vi "TagBus_Initialize_Map Data Type.vi"(11 "Value":variant) -> (3 "data type":T1)   [LabVIEW 2015, in "TagBus.lvclass"]
uses:
  TagBus.lvclass
  <vilib>/NI/Tag Bus/tag/Data Type.ctl
  <vilib>/Utility/Data Type/NI_Data Type.lvlib
  <vilib>/NI/Tag Bus/tag/tag descriptor.lvclass
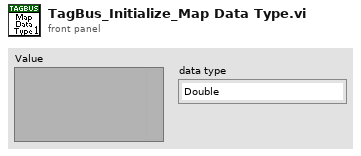
[diagram p1: front panel]
types:
  T1 = typedef "tag bus.lvlib/tag descriptor.lvclass/Data Type.ctl" = enum16{"Double", "Single", "I64", "I32", "I16", "I8", "U64", "U32", "U16", "U8", "Boolean", "String", "Array of Double", "Array of Single", "Array of I64", "Array of I32", "Array of I16", "Array of I8", "Array of U64", "Array of U32", "Array of U16", "Array of U8", "Array of Boolean", "Array of String"}
  T2 = typedef "NI_Data Type.lvlib/Data Type.ctl" = enum8{"Invalid Type", "Void", "I8", "I16", "I32", "I64", "U8", "U16", "U32", "U64", "Single Float", "Double Float", "Extended Float", "Single Complex", "Double Complex", "Extended Complex", "Enum U8", "Enum U16", "Enum U32", "Enum U64", "Single Float With Unit", "Double Float With Unit", "Extended Float With Unit", "Single Complex with Unit", "Double Complex with Unit", "Extended Complex with Unit", "Boolean", "String", "Path", "Picture", "Tag", "Array", "Cluster", "Variant", "LV Variant", "Waveform", "Timestamp", "Digital Waveform", "Digital Data", "ExpressData", "Refnum", "External Data", "VI", "Poly VI", "LabVIEW Class Instance", "Fixed Point"}
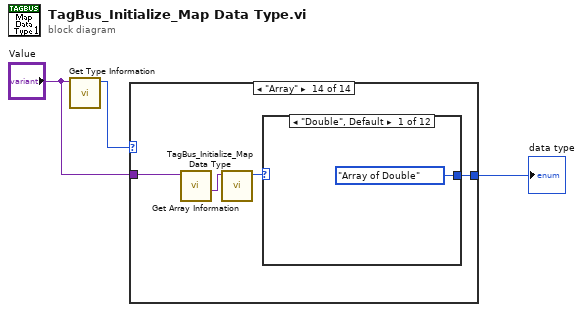
[diagram p0: block diagram]
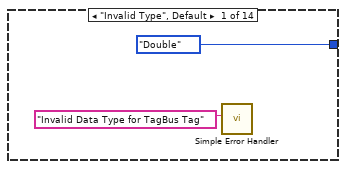
[diagram p2: hidden frame]
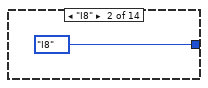
[diagram p3: hidden frame]
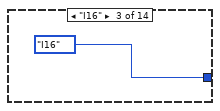
[diagram p4: hidden frame]
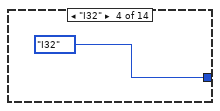
[diagram p5: hidden frame]
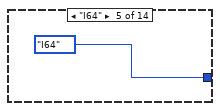
[diagram p6: hidden frame]
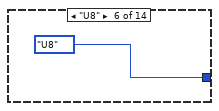
[diagram p7: hidden frame]
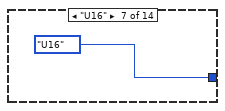
[diagram p8: hidden frame]
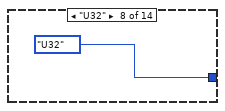
[diagram p9: hidden frame]
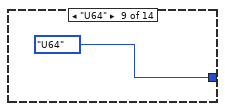
[diagram p10: hidden frame]
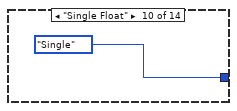
[diagram p11: hidden frame]
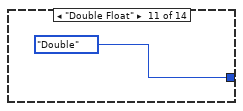
[diagram p12: hidden frame]
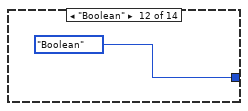
[diagram p13: hidden frame]
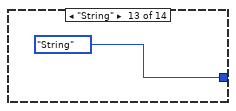
[diagram p14: hidden frame]
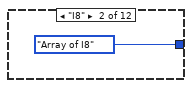
[diagram p15: hidden frame]
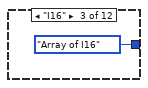
[diagram p16: hidden frame]
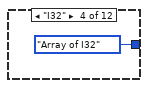
[diagram p17: hidden frame]
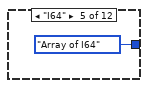
[diagram p18: hidden frame]
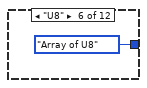
[diagram p19: hidden frame]
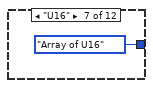
[diagram p20: hidden frame]
diagram:
  n1 = call <vilib>:"Get Type Information.vi"("Variant"="Value") -> ("Type"=w3:T2)  [unwired: 6 in, 4 out]
  n2 = case shown="\"Array\"" w3 {
    tunnel: [Data_Type."Double" ("data type") Data_Type."I8" ("data type") Data_Type."I16" ("data type") Data_Type."I32" ("data type") Data_Type."I64" ("data type") Data_Type."U8" ("data type") Data_Type."U16" ("data type") Data_Type."U32" ("data type") Data_Type."U64" ("data type") Data_Type."Single" ("data type") Data_Type."Double" ("data type") Data_Type."Boolean" ("data type") Data_Type."String" ("data type") w20] -> w1
    tunnel: "Value" -> [_ _ _ _ _ _ _ _ _ _ _ _ _ w21]
    frame "Invalid Type", Default {
      n3 = call <vilib>:"Simple Error Handler.vi"("error source (\" \")"="Invalid Data Type for TagBus Tag" ("error source (\" \")")) -> ()  [unwired: 4 in, 5 out]
    }
    frame "I8" {
    }
    frame "I16" {
    }
    frame "I32" {
    }
    frame "I64" {
    }
    frame "U8" {
    }
    frame "U16" {
    }
    frame "U32" {
    }
    frame "U64" {
    }
    frame "Single Float" {
    }
    frame "Double Float" {
    }
    frame "Boolean" {
    }
    frame "String" {
    }
    frame "Array" {
      n4 = call <vilib>:"Get Array Information.vi"("Variant"=w21) -> ("Array Element Data Type"=w19:variant)  [unwired: 7 in, 3 out]
      n5 = call "TagBus_Initialize_Map Data Type.vi"("Value"=w19) -> ("data type"=w18:T1)  [unwired: 10 in]
      n6 = case shown="\"Double\", Default" w18 {
        tunnel: [Data_Type."Array of Double" ("data type") Data_Type."Array of I8" ("data type") Data_Type."Array of I16" ("data type") Data_Type."Array of I32" ("data type") Data_Type."Array of I64" ("data type") Data_Type."Array of U8" ("data type") Data_Type."Array of U16" ("data type") Data_Type."Array of U32" ("data type") Data_Type."Array of U64" ("data type") Data_Type."Array of Boolean" ("data type") Data_Type."Array of Single" ("data type") Data_Type."Array of String" ("data type")] -> w20
        frame "Double", Default {
        }
        frame "I8" {
        }
        frame "I16" {
        }
        frame "I32" {
        }
        frame "I64" {
        }
        frame "U8" {
        }
        frame "U16" {
        }
        frame "U32" {
        }
        frame "U64" {
        }
        frame "Boolean" {
        }
        frame "Single" {
        }
        frame "String" {
        }
      }
    }
  }
  "data type" <- w1
